vi "main.vi"() -> ()   [LabVIEW 2023] (continued)
8        68\t00\t97\tCC\t00\t15\t39\t2B\r\n       342  18F120F0   00000004    8        2B\t75\t60\tB1\tB0\t01\tFF\tFF\r\n       341  18F11FF0   00000004    8        FF\t3F\t90\t68\t88\t1B\t10\tBC\r\n       332  1FFFFFFF   00000004    8        00\t00\tFF\tFF\tFF\tFF\tFF\tFF\r\n       323  0CF102A7   00000004    8        30\t75\tE0\t2E\t80\tFF\tFF\tFD\r\n       323  0CF101A7   00000004    8        68\t00\t97\tCC\t00\t15\t39\t2A\r\n       322  1FFFFFFF   00000004    8        00\t20\tFF\tFF\tFF\tFF\tFF\tFF\r\n       312  1FFFFFFF   00000004    8        00\t20\tFF\tFF\tFF\tFF\tFF\tFF\r\n       303  0CF102A7   00000004    8        30\t75\tE0\t2E\t80\tFF\tFF\tFD\r\n       344  0CF103A7   00000004    8        17\t1F\t08\t60\tB1\t1F\t08\t3B\r\n       344  0CF102A7   00000004    8        30\t75\tE0\t2E\t80\tFF\tFF\tFD\r\n       343  0C3C4D4A   00000004    8        BE\tFF\tFF\t7F\t18\tFF\tFF\t3B\r\n       343  0CF101A7   00000004    8        68\t00\t97\tCC\t00\t15\t39\t2B\r\n       342  18F120F0   00000004    8        2B\t75\t60\tB1\tB0\t01\tFF\tFF\r\n       341  18F11FF0   00000004    8        FF\t3F\t90\t68\t88\t1B\t10\tBC\r\n       332  1FFFFFFF   00000004    8        00\t00\tFF\tFF\tFF\tFF\tFF\tFF\r\n       323  0CF102A7   00000004    8        30\t75\tE0\t2E\t80\tFF\tFF\tFD\r\n       323  0CF101A7   00000004    8        68\t00\t97\tCC\t00\t15\t39\t2A\r\n       322  1FFFFFFF   00000004    8        00\t20\tFF\tFF\tFF\tFF\tFF\tFF\r\n       312  1FFFFFFF   00000004    8        00\t20\tFF\tFF\tFF\tFF\tFF\tFF\r\n       345  0CF104A7   00000004    8        F0\t60\t22\tFC\tFF\tFF\tFF\t3B\r\n       344  0CF103A7   00000004    8        17\t1F\t08\t60\tB1\t1F\t08\t3B\r\n       344  0CF102A7   00000004    8        30\t75\tE0\t2E\t80\tFF\tFF\tFD\r\n       343  0C3C4D4A   00000004    8        BE\tFF\tFF\t7F\t18\tFF\tFF\t3B\r\n       343  0CF101A7   00000004    8        68\t00\t97\tCC\t00\t15\t39\t2B\r\n       342  18F120F0   00000004    8        2B\t75\t60\tB1\tB0\t01\tFF\tFF\r\n       341  18F11FF0   00000004    8        FF\t3F\t90\t68\t88\t1B\t10\tBC\r\n       332  1FFFFFFF   00000004    8        00\t00\tFF\tFF\tFF\tFF\tFF\tFF\r\n       323  0CF102A7   00000004    8        30\t75\tE0\t2E\t80\tFF\tFF\tFD\r\n       323  0CF101A7   00000004    8        68\t00\t97\tCC\t00\t15\t39\t2A\r\n       322  1FFFFFFF   00000004    8        00\t20\tFF\tFF\tFF\tFF\tFF\tFF\r\n       345  18F106A7   00000004    8        00\tF7\tFF\tFF\tFF\tFF\tFF\t77\r\n       345  0CF104A7   00000004    8        F0\t60\t22\tFC\tFF\tFF\tFF\t3B\r\n       344  0CF103A7   00000004    8        17\t1F\t08\t60\tB1\t1F\t08\t3B\r\n       344  0CF102A7   00000004    8        30\t75\tE0\t2E\t80\tFF\tFF\tFD\r\n       343  0C3C4D4A   00000004    8        BE\tFF\tFF\t7F\t18\tFF\tFF\t3B\r\n       343  0CF101A7   00000004    8        68\t00\t97\tCC\t00\t15\t39\t2B\r\n       342  18F120F0   00000004    8        2B\t75\t60\tB1\tB0\t01\tFF\tFF\r\n       341  18F11FF0   00000004    8        FF\t3F\t90\t68\t88\t1B\t10\tBC\r\n       332  1FFFFFFF   00000004    8        00\t00\tFF\tFF\tFF\tFF\tFF\tFF\r\n       323  0CF102A7   00000004    8        30\t75\tE0\t2E\t80\tFF\tFF\tFD\r\n       323  0CF101A7   00000004    8        68\t00\t97\tCC\t00\t15\t39\t2A\r\n       346  18F121F0   00000004    8        09\t16\t00\t00\tFF\tFF\tB0\t01\r\n       345  18F106A7   00000004    8        00\tF7\tFF\tFF\tFF\tFF\tFF\t77\r\n       345  0CF104A7   00000004    8        F0\t60\t22\tFC\tFF\tFF\tFF\t3B\r\n       344  0CF103A7   00000004    8        17\t1F\t08\t60\tB1\t1F\t08\t3B\r\n       344  0CF102A7   00000004    8        30\t75\tE0\t2E\t80\tFF\tFF\tFD\r\n       343  0C3C4D4A   00000004    8        BE\tFF\tFF\t7F\t18\tFF\tFF\t3B\r\n       343  0CF101A7   00000004    8        68\t00\t97\tCC\t00\t15\t39\t2B\r\n       342  18F120F0   00000004    8        2B\t75\t60\tB1\tB0\t01\tFF\tFF\r\n       341  18F11FF0   00000004    8        FF\t3F\t90\t68\t88\t1B\t10\tBC\r\n       332  1FFFFFFF   00000004    8        00\t00\tFF\tFF\tFF\tFF\tFF\tFF\r\n       323  0CF102A7   00000004    8        30\t75\tE0\t2E\t80\tFF\tFF\tFD\r\n       347  1FFFFFFF   00000004    8        00\t00\tFF\tFF\tFF\tFF\tFF\tFF\r\n       346  18F121F0   00000004    8        09\t16\t00\t00\tFF\tFF\tB0\t01\r\n       345  18F106A7   00000004    8        00\tF7\tFF\tFF\tFF\tFF\tFF\t77\r\n       345  0CF104A7   00000004    8        F0\t60\t22\tFC\tFF\tFF\tFF\t3B\r\n       344  0CF103A7   00000004    8        17\t1F\t08\t60\tB1\t1F\t08\t3B\r\n       344  0CF102A7   00000004    8        30\t75\tE0\t2E\t80\tFF\tFF\tFD\r\n       343  0C3C4D4A   00000004    8        BE\tFF\tFF\t7F\t18\tFF\tFF\t3B\r\n       343  0CF101A7   00000004    8        68\t00\t97\tCC\t00\t15\t39\t2B\r\n       342  18F120F0   00000004    8        2B\t75\t60\tB1\tB0\t01\tFF\tFF\r\n       341  18F11FF0   00000004    8        FF\t3F\t90\t68\t88\t1B\t10\tBC\r\n       332  1FFFFFFF   00000004    8        00\t00\tFF\tFF\tFF\tFF\tFF\tFF\r\n       352  1FFFFFFF   00000004    8        00\t00\tFF\tFF\tFF\tFF\tFF\tFF\r\n       347  1FFFFFFF   00000004    8        00\t00\tFF\tFF\tFF\tFF\tFF\tFF\r\n       346  18F121F0   00000004    8        09\t16\t00\t00\tFF\tFF\tB0\t01\r\n       345  18F106A7   00000004    8        00\tF7\tFF\tFF\tFF\tFF\tFF\t77\r\n       345  0CF104A7   00000004    8        F0\t60\t22\tFC\tFF\tFF\tFF\t3B\r\n       344  0CF103A7   00000004    8        17\t1F\t08\t60\tB1\t1F\t08\t3B\r\n       344  0CF102A7   00000004    8        30\t75\tE0\t2E\t80\tFF\tFF\tFD\r\n       343  0C3C4D4A   00000004    8        BE\tFF\tFF\t7F\t18\tFF\tFF\t3B\r\n       343  0CF101A7   00000004    8        68\t00\t97\tCC\t00\t15\t39\t2B\r\n       342  18F120F0   00000004    8        2B\t75\t60\tB1\tB0\t01\tFF\tFF\r\n       341  18F11FF0   00000004    8        FF\t3F\t90\t68\t88\t1B\t10\tBC\r\n       362  1FFFFFFF   00000004    8        00\t00\tFF\tFF\tFF\tFF\tFF\tFF\r\n       352  1FFFFFFF   00000004    8        00\t00\tFF\tFF\tFF\tFF\tFF\tFF\r\n       347  1FFFFFFF   00000004    8        00\t00\tFF\tFF\tFF\tFF\tFF\tFF\r\n       346  18F121F0   00000004    8        09\t16\t00\t00\tFF\tFF\tB0\t01\r\n       345  18F106A7   00000004    8        00\tF7\tFF\tFF\tFF\tFF\tFF\t77\r\n       345  0CF104A7   00000004    8        F0\t60\t22\tFC\tFF\tFF\tFF\t3B\r\n       344  0CF103A7   00000004    8        17\t1F\t08\t60\tB1\t1F\t08\t3B\r\n       344  0CF102A7   00000004    8        30\t75\tE0\t2E\t80\tFF\tFF\tFD\r\n       343  0C3C4D4A   00000004    8        BE\tFF\tFF\t7F\t18\tFF\tFF\t3B\r\n       343  0CF101A7   00000004    8        68\t00\t97\tCC\t00\t15\t39\t2B\r\n       342  18F120F0   00000004    8        2B\t75\t60\tB1\tB0\t01\tFF\tFF\r\n       363  0CF101A7   00000004    8        68\t00\t97\tCC\t00\t15\t39\t2C\r\n       362  1FFFFFFF   00000004    8        00\t00\tFF\tFF\tFF\tFF\tFF\tFF\r\n       352  1FFFFFFF   00000004    8        00\t00\tFF\tFF\tFF\tFF\tFF\tFF\r\n       347  1FFFFFFF   00000004    8        00\t00\tFF\tFF\tFF\tFF\tFF\tFF\r\n       346  18F121F0   00000004    8        09\t16\t00\t00\tFF\tFF\tB0\t01\r\n       345  18F106A7   00000004    8        00\tF7\tFF\tFF\tFF\tFF\tFF\t77\r\n       345  0CF104A7   00000004    8        F0\t60\t22\tFC\tFF\tFF\tFF\t3B\r\n       344  0CF103A7   00000004    8        17\t1F\t08\t60\tB1\t1F\t08\t3B\r\n       344  0CF102A7   00000004    8        30\t75\tE0\t2E\t80\tFF\tFF\tFD\r\n       343  0C3C4D4A   00000004    8        BE\tFF\tFF\t7F\t18\tFF\tFF\t3B\r\n       343  0CF101A7   00000004    8        68\t00\t97\tCC\t00\t15\t39\t2B\r\n       363  0CF102A7   00000004    8        30\t75\tE0\t2E\t80\tFF\tFF\tFD\r\n       363  0CF101A7   00000004    8        68\t00\t97\tCC\t00\t15\t39\t2C\r\n       362  1FFFFFFF   00000004    8        00\t00\tFF\tFF\tFF\tFF\tFF\tFF\r\n       352  1FFFFFFF   00000004    8        00\t00\tFF\tFF\tFF\tFF\tFF\tFF\r\n       347  1FFFFFFF   00000004    8        00\t00\tFF\tFF\tFF\tFF\tFF\tFF\r\n       346  18F121F0   00000004    8        09\t16\t00\t00\tFF\tFF\tB0\t01\r\n       345  18F106A7   00000004    8        00\tF7\tFF\tFF\tFF\tFF\tFF\t77\r\n       345  0CF104A7   00000004    8        F0\t60\t22\tFC\tFF\tFF\tFF\t3B\r\n       344  0CF103A7   00000004    8        17\t1F\t08\t60\tB1\t1F\t08\t3B\r\n       344  0CF102A7   00000004    8        30\t75\tE0\t2E\t80\tFF\tFF\tFD\r\n       343  0C3C4D4A   00000004    8        BE\tFF\tFF\t7F\t18\tFF\tFF\t3B\r\n       372  1FFFFFFF   00000004    8        00\t20\tFF\tFF\tFF\tFF\tFF\tFF\r\n       363  0CF102A7   00000004    8        30\t75\tE0\t2E\t80\tFF\tFF\tFD\r\n       363  0CF101A7   00000004    8        68\t00\t97\tCC\t00\t15\t39\t2C\r\n       362  1FFFFFFF   00000004    8        00\t00\tFF\tFF\tFF\tFF\tFF\tFF\r\n       352  1FFFFFFF   00000004    8        00\t00\tFF\tFF\tFF\tFF\tFF\tFF\r\n       347  1FFFFFFF   00000004    8        00\t00\tFF\tFF\tFF\tFF\tFF\tFF\r\n       346  18F121F0   00000004    8        09\t16\t00\t00\tFF\tFF\tB0\t01\r\n       345  18F106A7   00000004    8        00\tF7\tFF\tFF\tFF\tFF\tFF\t77\r\n       345  0CF104A7   00000004    8        F0\t60\t22\tFC\tFF\tFF\tFF\t3B\r\n       344  0CF103A7   00000004    8        17\t1F\t08\t60\tB1\t1F\t08\t3B\r\n       344  0CF102A7   00000004    8        30\t75\tE0\t2E\t80\tFF\tFF\tFD\r\n       382  1FFFFFFF   00000004    8        00\t00\tFF\tFF\tFF\tFF\tFF\tFF\r\n       372  1FFFFFFF   00000004    8        00\t20\tFF\tFF\tFF\tFF\tFF\tFF\r\n       363  0CF102A7   00000004    8        30\t75\tE0\t2E\t80\tFF\tFF\tFD\r\n       363  0CF101A7   00000004    8        68\t00\t97\tCC\t00\t15\t39\t2C\r\n       362  1FFFFFFF   00000004    8        00\t00\tFF\tFF\tFF\tFF\tFF\tFF\r\n       352  1FFFFFFF   00000004    8        00\t00\tFF\tFF\tFF\tFF\tFF\tFF\r\n       347  1FFFFFFF   00000004    8        00\t00\tFF\tFF\tFF\tFF\tFF\tFF\r\n       346  18F121F0   00000004    8        09\t16\t00\t00\tFF\tFF\tB0\t01\r\n       345  18F106A7   00000004    8        00\tF7\tFF\tFF\tFF\tFF\tFF\t77\r\n       345  0CF104A7   00000004    8        F0\t60\t22\tFC\tFF\tFF\tFF\t3B\r\n       344  0CF103A7   00000004    8        17\t1F\t08\t60\tB1\t1F\t08\t3B\r\n       383  0CF101A7   00000004    8        68\t00\t97\tCC\t00\t15\t39\t2D\r\n       382  1FFFFFFF   00000004    8        00\t00\tFF\tFF\tFF\tFF\tFF\tFF\r\n       372  1FFFFFFF   00000004    8        00\t20\tFF\tFF\tFF\tFF\tFF\tFF\r\n       363  0CF102A7   00000004    8        30\t75\tE0\t2E\t80\tFF\tFF\tFD\r\n       363  0CF101A7   00000004    8        68\t00\t97\tCC\t00\t15\t39\t2C\r\n       362  1FFFFFFF   00000004    8        00\t00\tFF\tFF\tFF\tFF\tFF\tFF\r\n       352  1FFFFFFF   00000004    8        00\t00\tFF\tFF\tFF\tFF\tFF\tFF\r\n       347  1FFFFFFF   00000004    8        00\t00\tFF\tFF\tFF\tFF\tFF\tFF\r\n       346  18F121F0   00000004    8        09\t16\t00\t00\tFF\tFF\tB0\t01\r\n       345  18F106A7   00000004    8        00\tF7\tFF\tFF\tFF\tFF\tFF\t77\r\n       345  0CF104A7   00000004    8        F0\t60\t22\tFC\tFF\tFF\tFF\t3B\r\n       383  0CF102A7   00000004    8        30\t75\tE0\t2E\t80\tFF\tFF\tFD\r\n       383  0CF101A7   00000004    8        68\t00\t97\tCC\t00\t15\t39\t2D\r\n       382  1FFFFFFF   00000004    8        00\t00\tFF\tFF\tFF\tFF\tFF\tFF\r\n       372  1FFFFFFF   00000004    8        00\t20\tFF\tFF\tFF\tFF\tFF\tFF\r\n       363  0CF102A7   00000004    8        30\t75\tE0\t2E\t80\tFF\tFF\tFD\r\n       363  0CF101A7   00000004    8        68\t00\t97\tCC\t00\t15\t39\t2C\r\n       362  1FFFFFFF   00000004    8        00\t00\tFF\tFF\tFF\tFF\tFF\tFF\r\n       352  1FFFFFFF   00000004    8        00\t00\tFF\tFF\tFF\tFF\tFF\tFF\r\n       347  1FFFFFFF   00000004    8        00\t00\tFF\tFF\tFF\tFF\tFF\tFF\r\n       346  18F121F0   00000004    8        09\t16\t00\t00\tFF\tFF\tB0\t01\r\n       345  18F106A7   00000004    8        00\tF7\tFF\tFF\tFF\tFF\tFF\t77\r\n       392  1FFFFFFF   00000004    8        00\t00\tFF\tFF\tFF\tFF\tFF\tFF\r\n       383  0CF102A7   00000004    8        30\t75\tE0\t2E\t80\tFF\tFF\tFD\r\n       383  0CF101A7   00000004    8        68\t00\t97\tCC\t00\t15\t39\t2D\r\n       382  1FFFFFFF   00000004    8        00\t00\tFF\tFF\tFF\tFF\tFF\tFF\r\n       372  1FFFFFFF   00000004    8        00\t20\tFF\tFF\tFF\tFF\tFF\tFF\r\n       363  0CF102A7   00000004    8        30\t75\tE0\t2E\t80\tFF\tFF\tFD\r\n       363  0CF101A7   00000004    8        68\t00\t97\tCC\t00\t15\t39\t2C\r\n       362  1FFFFFFF   00000004    8        00\t00\tFF\tFF\tFF\tFF\tFF\tFF\r\n       352  1FFFFFFF   00000004    8        00\t00\tFF\tFF\tFF\tFF\tFF\tFF\r\n       347  1FFFFFFF   00000004    8        00\t00\tFF\tFF\tFF\tFF\tFF\tFF\r\n       346  18F121F0   00000004    8        09\t16\t00\t00\tFF\tFF\tB0\t01\r\n       393  18F106A7   00000004    8        00\tF7\tFF\tFF\tFF\tFF\tFF\t78\r\n       392  1FFFFFFF   00000004    8        00\t00\tFF\tFF\tFF\tFF\tFF\tFF\r\n       383  0CF102A7   00000004    8        30\t75\tE0\t2E\t80\tFF\tFF\tFD\r\n       383  0CF101A7   00000004    8        68\t00\t97\tCC\t00\t15\t39\t2D\r\n       382  1FFFFFFF   00000004    8        00\t00\tFF\tFF\tFF\tFF\tFF\tFF\r\n       372  1FFFFFFF   00000004    8        00\t20\tFF\tFF\tFF\tFF\tFF\tFF\r\n       363  0CF102A7   00000004    8        30\t75\tE0\t2E\t80\tFF\tFF\tFD\r\n       363  0CF101A7   00000004    8        68\t00\t97\tCC\t00\t15\t39\t2C\r\n       362  1FFFFFFF   00000004    8        00\t00\tFF\tFF\tFF\tFF\tFF\tFF\r\n       352  1FFFFFFF   00000004    8        00\t00\tFF\tFF\tFF\tFF\tFF\tFF\r\n       347  1FFFFFFF   00000004    8        00\t00\tFF\tFF\tFF\tFF\tFF\tFF\r\n       402  1FFFFFFF   00000004    8        00\t00\tFF\tFF\tFF\tFF\tFF\tFF\r\n       393  18F106A7   00000004    8        00\tF7\tFF\tFF\tFF\tFF\tFF\t78\r\n       392  1FFFFFFF   00000004    8        00\t00\tFF\tFF\tFF\tFF\tFF\tFF\r\n       383  0CF102A7   00000004    8        30\t75\tE0\t2E\t80\tFF\tFF\tFD\r\n       383  0CF101A7   00000004    8        68\t00\t97\tCC\t00\t15\t39\t2D\r\n       382  1FFFFFFF   00000004    8        00\t00\tFF\tFF\tFF\tFF\tFF\tFF\r\n       372  1FFFFFFF   00000004    8        00\t20\tFF\tFF\tFF\tFF\tFF\tFF\r\n       363  0CF102A7   00000004    8        30\t75\tE0\t2E\t80\tFF\tFF\tFD\r\n       363  0CF101A7   00000004    8        68\t00\t97\tCC\t00\t15\t39\t2C\r\n       362  1FFFFFFF   00000004    8        00\t00\tFF\tFF\tFF\tFF\tFF\tFF\r\n       352  1FFFFFFF   00000004    8        00\t00\tFF\tFF\tFF\tFF\tFF\tFF\r\n       403  0CF101A7   00000004    8        68\t00\t97\tCC\t00\t15\t39\t2E\r\n       402  1FFFFFFF   00000004    8        00\t00\tFF\tFF\tFF\tFF\tFF\tFF\r\n       393  18F106A7   00000004    8        00\tF7\tFF\tFF\tFF\tFF\tFF\t78\r\n       392  1FFFFFFF   00000004    8        00\t00\tFF\tFF\tFF\tFF\tFF\tFF\r\n       383  0CF102A7   00000004    8        30\t75\tE0\t2E\t80\tFF\tFF\tFD\r\n       383  0CF101A7   00000004    8        68\t00\t97\tCC\t00\t15\t39\t2D\r\n       382  1FFFFFFF   00000004    8        00\t00\tFF\tFF\tFF\tFF\tFF\tFF\r\n       372  1FFFFFFF   00000004    8        00\t20\tFF\tFF\tFF\tFF\tFF\tFF\r\n       363  0CF102A7   00000004    8        30\t75\tE0\t2E\t80\tFF\tFF\tFD\r\n       363  0CF101A7   00000004    8        68\t00\t97\tCC\t00\t15\t39\t2C\r\n       362  1FFFFFFF   00000004    8        00\t00\tFF\tFF\tFF\tFF\tFF\tFF\r\n       403  0CF102A7   00000004    8        30\t75\tE0\t2E\t80\tFF\tFF\tFD\r\n       403  0CF101A7   00000004    8        68\t00\t97\tCC\t00\t15\t39\t2E\r\n       402  1FFFFFFF   00000004    8        00\t00\tFF\tFF\tFF\tFF\tFF\tFF\r\n       393  18F106A7   00000004    8        00\tF7\tFF\tFF\tFF\tFF\tFF\t78\r\n       392  1FFFFFFF   00000004    8        00\t00\tFF\tFF\tFF\tFF\tFF\tFF\r\n       383  0CF102A7   00000004    8        30\t75\tE0\t2E\t80\tFF\tFF\tFD\r\n       383  0CF101A7   00000004    8        68\t00\t97\tCC\t00\t15\t39\t2D\r\n       382  1FFFFFFF   00000004    8        00\t00\tFF\tFF\tFF\tFF\tFF\tFF\r\n       372  1FFFFFFF   00000004    8        00\t20\tFF\tFF\tFF\tFF\tFF\tFF\r\n       363  0CF102A7   00000004    8        30\t75\tE0\t2E\t80\tFF\tFF\tFD\r\n       363  0CF101A7   00000004    8        68\t00\t97\tCC\t00\t15\t39\t2C\r\n       412  1FFFFFFF   00000004    8        00\t20\tFF\tFF\tFF\tFF\tFF\tFF\r\n       403  0CF102A7   00000004    8        30\t75\tE0\t2E\t80\tFF\tFF\tFD\r\n       403  0CF101A7   00000004    8        68\t00\t97\tCC\t00\t15\t39\t2E\r\n       402  1FFFFFFF   00000004    8        00\t00\tFF\tFF\tFF\tFF\tFF\tFF\r\n       393  18F106A7   00000004    8        00\tF7\tFF\tFF\tFF\tFF\tFF\t78\r\n       392  1FFFFFFF   00000004    8        00\t00\tFF\tFF\tFF\tFF\tFF\tFF\r\n       383  0CF102A7   00000004    8        30\t75\tE0\t2E\t80\tFF\tFF\tFD\r\n       383  0CF101A7   00000004    8        68\t00\t97\tCC\t00\t15\t39\t2D\r\n       382  1FFFFFFF   00000004    8        00\t00\tFF\tFF\tFF\tFF\tFF\tFF\r\n       372  1FFFFFFF   00000004    8        00\t20\tFF\tFF\tFF\tFF\tFF\tFF\r\n       363  0CF102A7   00000004    8        30\t75\tE0\t2E\t80\tFF\tFF\tFD\r\n       422  1FFFFFFF   00000004    8        00\t00\tFF\tFF\tFF\tFF\tFF\tFF\r\n       412  1FFFFFFF   00000004    8        00\t20\tFF\tFF\tFF\tFF\tFF\tFF\r\n       403  0CF102A7   00000004    8        30\t75\tE0\t2E\t80\tFF\tFF\tFD\r\n       403  0CF101A7   00000004    8        68\t00\t97\tCC\t00\t15\t39\t2E\r\n       402  1FFFFFFF   00000004    8        00\t00\tFF\tFF\tFF\tFF\tFF\tFF\r\n       393  18F106A7   00000004    8        00\tF7\tFF\tFF\tFF\tFF\tFF\t78\r\n       392  1FFFFFFF   00000004    8        00\t00\tFF\tFF\tFF\tFF\tFF\tFF\r\n       383  0CF102A7   00000004    8        30\t75\tE0\t2E\t80\tFF\tFF\tFD\r\n       383  0CF101A7   00000004    8        68\t00\t97\tCC\t00\t15\t39\t2D\r\n       382  1FFFFFFF   00000004    8        00\t00\tFF\tFF\tFF\tFF\tFF\tFF\r\n       372  1FFFFFFF   00000004    8        00\t20\tFF\tFF\tFF\tFF\tFF\tFF\r\n       423  0CF101A7   00000004    8        68\t00\t97\tCC\t00\t15\t39\t2F\r\n       422  1FFFFFFF   00000004    8        00\t00\tFF\tFF\tFF\tFF\tFF\tFF\r\n       412  1FFFFFFF   00000004    8        00\t20\tFF\tFF\tFF\tFF\tFF\tFF\r\n       403  0CF102A7   00000004    8        30\t75\tE0\t2E\t80\tFF\tFF\tFD\r\n       403  0CF101A7   00000004    8        68\t00\t97\tCC\t00\t15\t39\t2E\r\n       402  1FFFFFFF   00000004    8        00\t00\tFF\tFF\tFF\tFF\tFF\tFF\r\n       393  18F106A7   00000004    8        00\tF7\tFF\tFF\tFF\tFF\tFF\t78\r\n       392  1FFFFFFF   00000004    8        00\t00\tFF\tFF\tFF\tFF\tFF\tFF\r\n       383  0CF102A7   00000004    8        30\t75\tE0\t2E\t80\tFF\tFF\tFD\r\n       383  0CF101A7   00000004    8        68\t00\t97\tCC\t00\t15\t39\t2D\r\n       382  1FFFFFFF   00000004    8        00\t00\tFF\tFF\tFF\tFF\tFF\tFF\r\n       423  0CF102A7   00000004    8        30\t75\tE0\t2E\t80\tFF\tFF\tFD\r\n       423  0CF101A7   00000004    8        68\t00\t97\tCC\t00\t15\t39\t2F\r\n       422  1FFFFFFF   00000004    8        00\t00\tFF\tFF\tFF\tFF\tFF\tFF\r\n       412  1FFFFFFF   00000004    8        00\t20\tFF\tFF\tFF\tFF\tFF\tFF\r\n       403  0CF102A7   00000004    8        30\t75\tE0\t2E\t80\tFF\tFF\tFD\r\n       403  0CF101A7   00000004    8        68\t00\t97\tCC\t00\t15\t39\t2E\r\n       402  1FFFFFFF   00000004    8        00\t00\tFF\tFF\tFF\tFF\tFF\tFF\r\n       393  18F106A7   00000004    8        00\tF7\tFF\tFF\tFF\tFF\tFF\t78\r\n       392  1FFFFFFF   00000004    8        00\t00\tFF\tFF\tFF\tFF\tFF\tFF\r\n       383  0CF102A7   00000004    8        30\t75\tE0\t2E\t80\tFF\tFF\tFD\r\n       383  0CF101A7   00000004    8        68\t00\t97\tCC\t00\t15\t39\t2D\r\n       432  1FFFFFFF   00000004    8        00\t00\tFF\tFF\tFF\tFF\tFF\tFF\r\n       423  0CF102A7   00000004    8        30\t75\tE0\t2E\t80\tFF\tFF\tFD\r\n       423  0CF101A7   00000004    8        68\t00\t97\tCC\t00\t15\t39\t2F\r\n       422  1FFFFFFF   00000004    8        00\t00\tFF\tFF\tFF\tFF\tFF\tFF\r\n       412  1FFFFFFF   00000004    8        00\t20\tFF\tFF\tFF\tFF\tFF\tFF\r\n       403  0CF102A7   00000004    8        30\t75\tE0\t2E\t80\tFF\tFF\tFD\r\n       403  0CF101A7   00000004    8        68\t00\t97\tCC\t00\t15\t39\t2E\r\n       402  1FFFFFFF   00000004    8        00\t00\tFF\tFF\tFF\tFF\tFF\tFF\r\n       393  18F106A7   00000004    8        00\tF7\tFF\tFF\tFF\tFF\tFF\t78\r\n       392  1FFFFFFF   00000004    8        00\t00\tFF\tFF\tFF\tFF\tFF\tFF\r\n       383  0CF102A7   00000004    8        30\t75\tE0\t2E\t80\tFF\tFF\tFD\r\n       441  18F11FF0   00000004    8        FF\t3F\t90\t68\t88\t1B\t10\tCC\r\n       432  1FFFFFFF   00000004    8        00\t00\tFF\tFF\tFF\tFF\tFF\tFF\r\n       423  0CF102A7   00000004    8        30\t75\tE0\t2E\t80\tFF\tFF\tFD\r\n       423  0CF101A7   00000004    8        68\t00\t97\tCC\t00\t15\t39\t2F\r\n       422  1FFFFFFF   00000004    8        00\t00\tFF\tFF\tFF\tFF\tFF\tFF\r\n       412  1FFFFFFF   00000004    8        00\t20\tFF\tFF\tFF\tFF\tFF\tFF\r\n       403  0CF102A7   00000004    8        30\t75\tE0\t2E\t80\tFF\tFF\tFD\r\n       403  0CF101A7   00000004    8        68\t00\t97\tCC\t00\t15\t39\t2E\r\n       402  1FFFFFFF   00000004    8        00\t00\tFF\tFF\tFF\tFF\tFF\tFF\r\n       393  18F106A7   00000004    8        00\tF7\tFF\tFF\tFF\tFF\tFF\t78\r\n       392  1FFFFFFF   00000004    8        00\t00\tFF\tFF\tFF\tFF\tFF\tFF\r\n       442  18F120F0   00000004    8        2B\t75\t60\tB1\tB0\t01\tFF\tFF\r\n       441  18F11FF0   00000004    8        FF\t3F\t90\t68\t88\t1B\t10\tCC\r\n       432  1FFFFFFF   00000004    8        00\t00\tFF\tFF\tFF\tFF\tFF\tFF\r\n       423  0CF102A7   00000004    8        30\t75\tE0\t2E\t80\tFF\tFF\tFD\r\n       423  0CF101A7   00000004    8        68\t00\t97\tCC\t00\t15\t39\t2F\r\n       422  1FFFFFFF   00000004    8        00\t00\tFF\tFF\tFF\tFF\tFF\tFF\r\n       412  1FFFFFFF   00000004    8        00\t20\tFF\tFF\tFF\tFF\tFF\tFF\r\n       403  0CF102A7   00000004    8        30\t75\tE0\t2E\t80\tFF\tFF\tFD\r\n       403  0CF101A7   00000004    8        68\t00\t97\tCC\t00\t15\t39\t2E\r\n       402  1FFFFFFF   00000004    8        00\t00\tFF\tFF\tFF\tFF\tFF\tFF\r\n       393  18F106A7   00000004    8        00\tF7\tFF\tFF\tFF\tFF\tFF\t78\r\n       443  0CF101A7   00000004    8        68\t00\t97\tCC\t00\t15\t39\t30\r\n       442  18F120F0   00000004    8        2B\t75\t60\tB1\tB0\t01\tFF\tFF\r\n       441  18F11FF0   00000004    8        FF\t3F\t90\t68\t88\t1B\t10\tCC\r\n       432  1FFFFFFF   00000004    8        00\t00\tFF\tFF\tFF\tFF\tFF\tFF\r\n       423  0CF102A7   00000004    8        30\t75\tE0\t2E\t80\tFF\tFF\tFD\r\n       423  0CF101A7   00000004    8        68\t00\t97\tCC\t00\t15\t39\t2F\r\n       422  1FFFFFFF   00000004    8        00\t00\tFF\tFF\tFF\tFF\tFF\tFF\r\n       412  1FFFFFFF   00000004    8        00\t20\tFF\tFF\tFF\tFF\tFF\tFF\r\n       403  0CF102A7   00000004    8        30\t75\tE0\t2E\t80\tFF\tFF\tFD\r\n       403  0CF101A7   00000004    8        68\t00\t97\tCC\t00\t15\t39\t2E\r\n       402  1FFFFFFF   00000004    8        00\t00\tFF\tFF\tFF\tFF\tFF\tFF\r\n       443  0C3C4D4A   00000004    8        BE\tFF\tFF\t7F\t18\tFF\tFF\t3C\r\n       443  0CF101A7   00000004    8        68\t00\t97\tCC\t00\t15\t39\t30\r\n       442  18F120F0   00000004    8        2B\t75\t60\tB1\tB0\t01\tFF\tFF\r\n       441  18F11FF0   00000004    8        FF\t3F\t90\t68\t88\t1B\t10\tCC\r\n       432  1FFFFFFF   00000004    8        00\t00\tFF\tFF\tFF\tFF\tFF\tFF\r\n       423  0CF102A7   00000004    8        30\t75\tE0\t2E\t80\tFF\tFF\tFD\r\n       423  0CF101A7   00000004    8        68\t00\t97\tCC\t00\t15\t39\t2F\r\n       422  1FFFFFFF   00000004    8        00\t00\tFF\tFF\tFF\tFF\tFF\tFF\r\n       412  1FFFFFFF   00000004    8        00\t20\tFF\tFF\tFF\tFF\tFF\tFF\r\n       403  0CF102A7   00000004    8        30\t75\tE0\t2E\t80\tFF\tFF\tFD\r\n       403  0CF101A7   00000004    8        68\t00\t97\tCC\t00\t15\t39\t2E\r\n       444  0CF102A7   00000004    8        30\t75\tE0\t2E\t80\tFF\tFF\tFD\r\n       443  0C3C4D4A   00000004    8        BE\tFF\tFF\t7F\t18\tFF\tFF\t3C\r\n       443  0CF101A7   00000004    8        68\t00\t97\tCC\t00\t15\t39\t30\r\n       442  18F120F0   00000004    8        2B\t75\t60\tB1\tB0\t01\tFF\tFF\r\n       441  18F11FF0   00000004    8        FF\t3F\t90\t68\t88\t1B\t10\tCC\r\n       432  1FFFFFFF   00000004    8        00\t00\tFF\tFF\tFF\tFF\tFF\tFF\r\n       423  0CF102A7   00000004    8        30\t75\tE0\t2E\t80\tFF\tFF\tFD\r\n       423  0CF101A7   00000004    8        68\t00\t97\tCC\t00\t15\t39\t2F\r\n       422  1FFFFFFF   00000004    8        00\t00\tFF\tFF\tFF\tFF\tFF\tFF\r\n       412  1FFFFFFF   00000004    8        00\t20\tFF\tFF\tFF\tFF\tFF\tFF\r\n       403  0CF102A7   00000004    8        30\t75\tE0\t2E\t80\tFF\tFF\tFD\r\n       444  0CF103A7   00000004    8        17\t1F\t08\t60\tB1\t1F\t08\t3C\r\n       444  0CF102A7   00000004    8        30\t75\tE0\t2E\t80\tFF\tFF\tFD\r\n       443  0C3C4D4A   00000004    8        BE\tFF\tFF\t7F\t18\tFF\tFF\t3C\r\n       443  0CF101A7   00000004    8        68\t00\t97\tCC\t00\t15\t39\t30\r\n       442  18F120F0   00000004    8        2B\t75\t60\tB1\tB0\t01\tFF\tFF\r\n       441  18F11FF0   00000004    8        FF\t3F\t90\t68\t88\t1B\t10\tCC\r\n       432  1FFFFFFF   00000004    8        00\t00\tFF\tFF\tFF\tFF\tFF\tFF\r\n       423  0CF102A7   00000004    8        30\t75\tE0\t2E\t80\tFF\tFF\tFD\r\n       423  0CF101A7   00000004    8        68\t00\t97\tCC\t00\t15\t39\t2F\r\n       422  1FFFFFFF   00000004    8        00\t00\tFF\tFF\tFF\tFF\tFF\tFF\r\n       412  1FFFFFFF   00000004    8        00\t20\tFF\tFF\tFF\tFF\tFF\tFF\r\n       445  0CF104A7   00000004    8        F0\t60\t22\tFC\tFF\tFF\tFF\t3C\r\n       444  0CF103A7   00000004    8        17\t1F\t08\t60\tB1\t1F\t08\t3C\r\n       444  0CF102A7   00000004    8        30\t75\tE0\t2E\t80\tFF\tFF\tFD\r\n       443  0C3C4D4A   00000004    8        BE\tFF\tFF\t7F\t18\tFF\tFF\t3C\r\n       443  0CF101A7   00000004    8        68\t00\t97\tCC\t00\t15\t39\t30\r\n       442  18F120F0   00000004    8        2B\t75\t60\tB1\tB0\t01\tFF\tFF\r\n       441  18F11FF0   00000004    8        FF\t3F\t90\t68\t88\t1B\t10\tCC\r\n       432  1FFFFFFF   00000004    8        00\t00\tFF\tFF\tFF\tFF\tFF\tFF\r\n       423  0CF102A7   00000004    8        30\t75\tE0\t2E\t80\tFF\tFF\tFD\r\n       423  0CF101A7   00000004    8        68\t00\t97\tCC\t00\t15\t39\t2F\r\n       422  1FFFFFFF   00000004    8        00\t00\tFF\tFF\tFF\tFF\tFF\tFF\r\n       445  18F106A7   00000004    8        00\tF7\tFF\tFF\tFF\tFF\tFF\t79\r\n       445  0CF104A7   00000004    8        F0\t60\t22\tFC\tFF\tFF\tFF\t3C\r\n       444  0CF103A7   00000004    8        17\t1F\t08\t60\tB1\t1F\t08\t3C\r\n       444  0CF102A7   00000004    8        30\t75\tE0\t2E\t80\tFF\tFF\tFD\r\n       443  0C3C4D4A   00000004    8        BE\tFF\tFF\t7F\t18\tFF\tFF\t3C\r\n       443  0CF101A7   00000004    8        68\t00\t97\tCC\t00\t15\t39\t30\r\n       442  18F120F0   00000004    8        2B\t75\t60\tB1\tB0\t01\tFF\tFF\r\n       441  18F11FF0   00000004    8        FF\t3F\t90\t68\t88\t1B\t10\tCC\r\n       432  1FFFFFFF   00000004    8        00\t00\tFF\tFF\tFF\tFF\tFF\tFF\r\n       423  0CF102A7   00000004    8        30\t75\tE0\t2E\t80\tFF\tFF\tFD\r\n       423  0CF101A7   00000004    8        68\t00\t97\tCC\t00\t15\t39\t2F\r\n       446  18F121F0   00000004    8        09\t16\t00\t00\tFF\tFF\tB0\t01\r\n       445  18F106A7   00000004    8        00\tF7\tFF\tFF\tFF\tFF\tFF\t79\r\n       445  0CF104A7   00000004    8        F0\t60\t22\tFC\tFF\tFF\tFF\t3C\r\n       444  0CF103A7   00000004    8        17\t1F\t08\t60\tB1\t1F\t08\t3C\r\n       444  0CF102A7   00000004    8        30\t75\tE0\t2E\t80\tFF\tFF\tFD\r\n       443  0C3C4D4A   00000004    8        BE\tFF\tFF\t7F\t18\tFF\tFF\t3C\r\n       443  0CF101A7   00000004    8        68\t00\t97\tCC\t00\t15\t39\t30\r\n       442  18F120F0   00000004    8        2B\t75\t60\tB1\tB0\t01\tFF\tFF\r\n       441  18F11FF0   00000004    8        FF\t3F\t90\t68\t88\t1B\t10\tCC\r\n       432  1FFFFFFF   00000004    8        00\t00\tFF\tFF\tFF\tFF\tFF\tFF\r\n       423  0CF102A7   00000004    8        30\t75\tE0\t2E\t80\tFF\tFF\tFD\r\n       447  1FFFFFFF   00000004    8        00\t00\tFF\tFF\tFF\tFF\tFF\tFF\r\n       446  18F121F0   00000004    8        09\t16\t00\t00\tFF\tFF\tB0\t01\r\n       445  18F106A7   00000004    8        00\tF7\tFF\tFF\tFF\tFF\tFF\t79\r\n       445  0CF104A7   00000004    8        F0\t60\t22\tFC\tFF\tFF\tFF\t3C\r\n       444  0CF103A7   00000004    8        17\t1F\t08\t60\tB1\t1F\t08\t3C\r\n       444  0CF102A7   00000004    8        30\t75\tE0\t2E\t80\tFF\tFF\tFD\r\n       443  0C3C4D4A   00000004    8        BE\tFF\tFF\t7F\t18\tFF\tFF\t3C\r\n       443  0CF101A7   00000004    8        68\t00\t97\tCC\t00\t15\t39\t30\r\n       442  18F120F0   00000004    8        2B\t75\t60\tB1\tB0\t01\tFF\tFF\r\n       441  18F11FF0   00000004    8        FF\t3F\t90\t68\t88\t1B\t10\tCC\r\n       432  1FFFFFFF   00000004    8        00\t00\tFF\tFF\tFF\tFF\tFF\tFF\r\n       452  1FFFFFFF   00000004    8        00\t20\tFF\tFF\tFF\tFF\tFF\tFF\r\n       447  1FFFFFFF   00000004    8        00\t00\tFF\tFF\tFF\tFF\tFF\tFF\r\n       446  18F121F0   00000004    8        09\t16\t00\t00\tFF\tFF\tB0\t01\r\n       445  18F106A7   00000004    8        00\tF7\tFF\tFF\tFF\tFF\tFF\t79\r\n       445  0CF104A7   00000004    8        F0\t60\t22\tFC\tFF\tFF\tFF\t3C\r\n       444  0CF103A7   00000004    8        17\t1F\t08\t60\tB1\t1F\t08\t3C\r\n       444  0CF102A7   00000004    8        30\t75\tE0\t2E\t80\tFF\tFF\tFD\r\n       443  0C3C4D4A   00000004    8        BE\tFF\tFF\t7F\t18\tFF\tFF\t3C\r\n       443  0CF101A7   00000004    8        68\t00\t97\tCC\t00\t15\t39\t30\r\n       442  18F120F0   00000004    8        2B\t75\t60\tB1\tB0\t01\tFF\tFF\r\n       441  18F11FF0   00000004    8        FF\t3F\t90\t68\t88\t1B\t10\tCC\r\n       462  1FFFFFFF   00000004    8        00\t00\tFF\tFF\tFF\tFF\tFF\tFF\r\n       452  1FFFFFFF   00000004    8        00\t20\tFF\tFF\tFF\tFF\tFF\tFF\r\n       447  1FFFFFFF   00000004    8        00\t00\tFF\tFF\tFF\tFF\tFF\tFF\r\n       446  18F121F0   00000004    8        09\t16\t00\t00\tFF\tFF\tB0\t01\r\n       445  18F106A7   00000004    8        00\tF7\tFF\tFF\tFF\tFF\tFF\t79\r\n       445  0CF104A7   00000004    8        F0\t60\t22\tFC\tFF\tFF\tFF\t3C\r\n       444  0CF103A7   00000004    8        17\t1F\t08\t60\tB1\t1F\t08\t3C\r\n       444  0CF102A7   00000004    8        30\t75\tE0\t2E\t80\tFF\tFF\tFD\r\n       443  0C3C4D4A   00000004    8        BE\tFF\tFF\t7F\t18\tFF\tFF\t3C\r\n       443  0CF101A7   00000004    8        68\t00\t97\tCC\t00\t15\t39\t30\r\n       442  18F120F0   00000004    8        2B\t75\t60\tB1\tB0\t01\tFF\tFF\r\n       463  0CF101A7   00000004    8        68\t00\t97\tCC\t00\t15\t39\t31\r\n       462  1FFFFFFF   00000004    8        00\t00\tFF\tFF\tFF\tFF\tFF\tFF\r\n       452  1FFFFFFF   00000004    8        00\t20\tFF\tFF\tFF\tFF\tFF\tFF\r\n       447  1FFFFFFF   00000004    8        00\t00\tFF\tFF\tFF\tFF\tFF\tFF\r\n       446  18F121F0   00000004    8        09\t16\t00\t00\tFF\tFF\tB0\t01\r\n       445  18F106A7   00000004    8        00\tF7\tFF\tFF\tFF\tFF\tFF\t79\r\n       445  0CF104A7   00000004    8        F0\t60\t22\tFC\tFF\tFF\tFF\t3C\r\n       444  0CF103A7   00000004    8        17\t1F\t08\t60\tB1\t1F\t08\t3C\r\n       444  0CF102A7   00000004    8        30\t75\tE0\t2E\t80\tFF\tFF\tFD\r\n       443  0C3C4D4A   00000004    8        BE\tFF\tFF\t7F\t18\tFF\tFF\t3C\r\n       443  0CF101A7   00000004    8        68\t00\t97\tCC\t00\t15\t39\t30\r\n       463  0CF102A7   00000004    8        30\t75\tE0\t2E\t80\tFF\tFF\tFD\r\n       463  0CF101A7   00000004    8        68\t00\t97\tCC\t00\t15\t39\t31\r\n       462  1FFFFFFF   00000004    8        00\t00\tFF\tFF\tFF\tFF\tFF\tFF\r\n       452  1FFFFFFF   00000004    8        00\t20\tFF\tFF\tFF\tFF\tFF\tFF\r\n       447  1FFFFFFF   00000004    8        00\t00\tFF\tFF\tFF\tFF\tFF\tFF\r\n       446  18F121F0   00000004    8        09\t16\t00\t00\tFF\tFF\tB0\t01\r\n       445  18F106A7   00000004    8        00\tF7\tFF\tFF\tFF\tFF\tFF\t79\r\n       445  0CF104A7   00000004    8        F0\t60\t22\tFC\tFF\tFF\tFF\t3C\r\n       444  0CF103A7   00000004    8        17\t1F\t08\t60\tB1\t1F\t08\t3C\r\n       444  0CF102A7   00000004    8        30\t75\tE0\t2E\t80\tFF\tFF\tFD\r\n       443  0C3C4D4A   00000004    8        BE\tFF\tFF\t7F\t18\tFF\tFF\t3C\r\n       472  1FFFFFFF   00000004    8        00\t20\tFF\tFF\tFF\tFF\tFF\tFF\r\n       463  0CF102A7   00000004    8        30\t75\tE0\t2E\t80\tFF\tFF\tFD\r\n       463  0CF101A7   00000004    8        68\t00\t97\tCC\t00\t15\t39\t31\r\n       462  1FFFFFFF   00000004    8        00\t00\tFF\tFF\tFF\tFF\tFF\tFF\r\n       452  1FFFFFFF   00000004    8        00\t20\tFF\tFF\tFF\tFF\tFF\tFF\r\n       447  1FFFFFFF   00000004    8        00\t00\tFF\tFF\tFF\tFF\tFF\tFF\r\n       446  18F121F0   00000004    8        09\t16\t00\t00\tFF\tFF\tB0\t01\r\n       445  18F106A7   00000004    8        00\tF7\tFF\tFF\tFF\tFF\tFF\t79\r\n       445  0CF104A7   00000004    8        F0\t60\t22\tFC\tFF\tFF\tFF\t3C\r\n       444  0CF103A7   00000004    8        17\t1F\t08\t60\tB1\t1F\t08\t3C\r\n       444  0CF102A7   00000004    8        30\t75\tE0\t2E\t80\tFF\tFF\tFD\r\n       482  1FFFFFFF   00000004    8        00\t20\tFF\tFF\tFF\tFF\tFF\tFF\r\n       472  1FFFFFFF   00000004    8        00\t20\tFF\tFF\tFF\tFF\tFF\tFF\r\n       463  0CF102A7   00000004    8        30\t75\tE0\t2E\t80\tFF\tFF\tFD\r\n       463  0CF101A7   00000004    8        68\t00\t97\tCC\t00\t15\t39\t31\r\n       462  1FFFFFFF   00000004    8        00\t00\tFF\tFF\tFF\tFF\tFF\tFF\r\n       452  1FFFFFFF   00000004    8        00\t20\tFF\tFF\tFF\tFF\tFF\tFF\r\n       447  1FFFFFFF   00000004    8        00\t00\tFF\tFF\tFF\tFF\tFF\tFF\r\n       446  18F121F0   00000004    8        09\t16\t00\t00\tFF\tFF\tB0\t01\r\n       445  18F106A7   00000004    8        00\tF7\tFF\tFF\tFF\tFF\tFF\t79\r\n       445  0CF104A7   00000004    8        F0\t60\t22\tFC\tFF\tFF\tFF\t3C\r\n       444  0CF103A7   00000004    8        17\t1F\t08\t60\tB1\t1F\t08\t3C\r\n       483  0CF101A7   00000004    8        68\t00\t97\tCC\t00\t15\t39\t32\r\n       482  1FFFFFFF   00000004    8        00\t20\tFF\tFF\tFF\tFF\tFF\tFF\r\n       472  1FFFFFFF   00000004    8        00\t20\tFF\tFF\tFF\tFF\tFF\tFF\r\n       463  0CF102A7   00000004    8        30\t75\tE0\t2E\t80\tFF\tFF\tFD\r\n       463  0CF101A7   00000004    8        68\t00\t97\tCC\t00\t15\t39\t31\r\n       462  1FFFFFFF   00000004    8        00\t00\tFF\tFF\tFF\tFF\tFF\tFF\r\n       452  1FFFFFFF   00000004    8        00\t20\tFF\tFF\tFF\tFF\tFF\tFF\r\n       447  1FFFFFFF   00000004    8        00\t00\tFF\tFF\tFF\tFF\tFF\tFF\r\n       446  18F121F0   00000004    8        09\t16\t00\t00\tFF\tFF\tB0\t01\r\n       445  18F106A7   00000004    8        00\tF7\tFF\tFF\tFF\tFF\tFF\t79\r\n       445  0CF104A7   00000004    8        F0\t60\t22\tFC\tFF\tFF\tFF\t3C\r\n       483  0CF102A7   00000004    8        30\t75\tE0\t2E\t80\tFF\tFF\tFD\r\n       483  0CF101A7   00000004    8        68\t00\t97\tCC\t00\t15\t39\t32\r\n       482  1FFFFFFF   00000004    8        00\t20\tFF\tFF\tFF\tFF\tFF\tFF\r\n       472  1FFFFFFF   00000004    8        00\t20\tFF\tFF\tFF\tFF\tFF\tFF\r\n       463  0CF102A7   00000004    8        30\t75\tE0\t2E\t80\tFF\tFF\tFD\r\n       463  0CF101A7   00000004    8        68\t00\t97\tCC\t00\t15\t39\t31\r\n       462  1FFFFFFF   00000004    8        00\t00\tFF\tFF\tFF\tFF\tFF\tFF\r\n       452  1FFFFFFF   00000004    8        00\t20\tFF\tFF\tFF\tFF\tFF\tFF\r\n       447  1FFFFFFF   00000004    8        00\t00\tFF\tFF\tFF\tFF\tFF\tFF\r\n       446  18F121F0   00000004    8        09\t16\t00\t00\tFF\tFF\tB0\t01\r\n       445  18F106A7   00000004    8        00\tF7\tFF\tFF\tFF\tFF\tFF\t79\r\n       492  1FFFFFFF   00000004    8        00\t00\tFF\tFF\tFF\tFF\tFF\tFF\r\n       483  0CF102A7   00000004    8        30\t75\tE0\t2E\t80\tFF\tFF\tFD\r\n       483  0CF101A7   00000004    8        68\t00\t97\tCC\t00\t15\t39\t32\r\n       482  1FFFFFFF   00000004    8        00\t20\tFF\tFF\tFF\tFF\tFF\tFF\r\n       472  1FFFFFFF   00000004    8        00\t20\tFF\tFF\tFF\tFF\tFF\tFF\r\n       463  0CF102A7   00000004    8        30\t75\tE0\t2E\t80\tFF\tFF\tFD\r\n       463  0CF101A7   00000004    8        68\t00\t97\tCC\t00\t15\t39\t31\r\n       462  1FFFFFFF   00000004    8        00\t00\tFF\tFF\tFF\tFF\tFF\tFF\r\n       452  1FFFFFFF   00000004    8        00\t20\tFF\tFF\tFF\tFF\tFF\tFF\r\n       447  1FFFFFFF   00000004    8        00\t00\tFF\tFF\tFF\tFF\tFF\tFF\r\n       446  18F121F0   00000004    8        09\t16\t00\t00\tFF\tFF\tB0\t01\r\n       493  18F106A7   00000004    8        00\tF7\tFF\tFF\tFF\tFF\tFF\t7A\r\n       492  1FFFFFFF   00000004    8        00\t00\tFF\tFF\tFF\tFF\tFF\tFF\r\n       483  0CF102A7   00000004    8        30\t75\tE0\t2E\t80\tFF\tFF\tFD\r\n       483  0CF101A7   00000004    8        68\t00\t97\tCC\t00\t15\t39\t32\r\n       482  1FFFFFFF   00000004    8        00\t20\tFF\tFF\tFF\tFF\tFF\tFF\r\n       472  1FFFFFFF   00000004    8        00\t20\tFF\tFF\tFF\tFF\tFF\tFF\r\n       463  0CF102A7   00000004    8        30\t75\tE0\t2E\t80\tFF\tFF\tFD\r\n       463  0CF101A7   00000004    8        68\t00\t97\tCC\t00\t15\t39\t31\r\n       462  1FFFFFFF   00000004    8        00\t00\tFF\tFF\tFF\tFF\tFF\tFF\r\n       452  1FFFFFFF   00000004    8        00\t20\tFF\tFF\tFF\tFF\tFF\tFF\r\n       447  1FFFFFFF   00000004    8        00\t00\tFF\tFF\tFF\tFF\tFF\tFF\r\n       502  1FFFFFFF   00000004    8        00\t20\tFF\tFF\tFF\tFF\tFF\tFF\r\n       493  18F106A7   00000004    8        00\tF7\tFF\tFF\tFF\tFF\tFF\t7A\r\n       492  1FFFFFFF   00000004    8        00\t00\tFF\tFF\tFF\tFF\tFF\tFF\r\n       483  0CF102A7   00000004    8        30\t75\tE0\t2E\t80\tFF\tFF\tFD\r\n       483  0CF101A7   00000004    8        68\t00\t97\tCC\t00\t15\t39\t32\r\n       482  1FFFFFFF   00000004    8        00\t20\tFF\tFF\tFF\tFF\tFF\tFF\r\n       472  1FFFFFFF   00000004    8        00\t20\tFF\tFF\tFF\tFF\tFF\tFF\r\n       463  0CF102A7   00000004    8        30\t75\tE0\t2E\t80\tFF\tFF\tFD\r\n       463  0CF101A7   00000004    8        68\t00\t97\tCC\t00\t15\t39\t31\r\n       462  1FFFFFFF   00000004    8        00\t00\tFF\tFF\tFF\tFF\tFF\tFF\r\n       452  1FFFFFFF   00000004    8        00\t20\tFF\tFF\tFF\tFF\tFF\tFF\r\n       503  0CF101A7   00000004    8        68\t00\t97\tCC\t00\t15\t39\t33\r\n       502  1FFFFFFF   00000004    8        00\t20\tFF\tFF\tFF\tFF\tFF\tFF\r\n       493  18F106A7   00000004    8        00\tF7\tFF\tFF\tFF\tFF\tFF\t7A\r\n       492  1FFFFFFF   00000004    8        00\t00\tFF\tFF\tFF\tFF\tFF\tFF\r\n       483  0CF102A7   00000004    8        30\t75\tE0\t2E\t80\tFF\tFF\tFD\r\n       483  0CF101A7   00000004    8        68\t00\t97\tCC\t00\t15\t39\t32\r\n       482  1FFFFFFF   00000004    8        00\t20\tFF\tFF\tFF\tFF\tFF\tFF\r\n       472  1FFFFFFF   00000004    8        00\t20\tFF\tFF\tFF\tFF\tFF\tFF\r\n       463  0CF102A7   00000004    8        30\t75\tE0\t2E\t80\tFF\tFF\tFD\r\n       463  0CF101A7   00000004    8        68\t00\t97\tCC\t00\t15\t39\t31\r\n       462  1FFFFFFF   00000004    8        00\t00\tFF\tFF\tFF\tFF\tFF\tFF\r\n       503  0CF102A7   00000004    8        30\t75\tE0\t2E\t80\tFF\tFF\tFD\r\n       503  0CF101A7   00000004    8        68\t00\t97\tCC\t00\t15\t39\t33\r\n       502  1FFFFFFF   00000004    8        00\t20\tFF\tFF\tFF\tFF\tFF\tFF\r\n       493  18F106A7   00000004    8        00\tF7\tFF\tFF\tFF\tFF\tFF\t7A\r\n       492  1FFFFFFF   00000004    8        00\t00\tFF\tFF\tFF\tFF\tFF\tFF\r\n       483  0CF102A7   00000004    8        30\t75\tE0\t2E\t80\tFF\tFF\tFD\r\n       483  0CF101A7   00000004    8        68\t00\t97\tCC\t00\t15\t39\t32\r\n       482  1FFFFFFF   00000004    8        00\t20\tFF\tFF\tFF\tFF\tFF\tFF\r\n       472  1FFFFFFF   00000004    8        00\t20\tFF\tFF\tFF\tFF\tFF\tFF\r\n       463 
